vi "Test Open or Create.vi"(11 "Test Case In":refnum<class "Test Open Xml.lvclass">) -> (0 "error out":errorcluster, 3 "Test Case Out":refnum<class "Test Open Xml.lvclass">)   [LabVIEW 2020, in "Test Open Xml.lvclass"]
uses:
  Test Open Xml.lvclass
  C:/Program Files/National Instruments/LabVIEW 2025/vi.lib/Astemes/LUnit/Test Case.lvclass
  <vilib>/Astemes/LUnit/Test Case.lvclass/Test Case.ctl
  2c4bb252-386c-45a5-bd4c-bbe84a65a97e.vi
  <vilib>/Astemes/LUnit/Core/LUnit Test Case/Private/Append Pass Result.vi
  <vilib>/Astemes/LUnit/Core/LUnit Test Case/Private/Append Fail Result.vi
  2c4bb252-386c-45a5-bd4c-bbe84a65a97e.vi/9c5d11cd-9439-4240-a1ee-d9baace9c924.vi
  <vilib>/Astemes/LUnit/Core/LUnit Test Case/Private/Run In UI.vi
  <vilib>/Utility/error.llb/Clear Errors.vi
  Source/Open Xml.lvlib
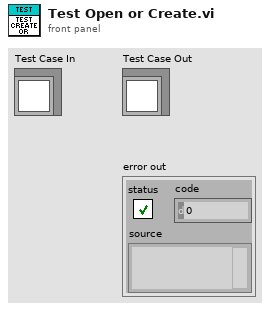
[diagram p1: front panel]
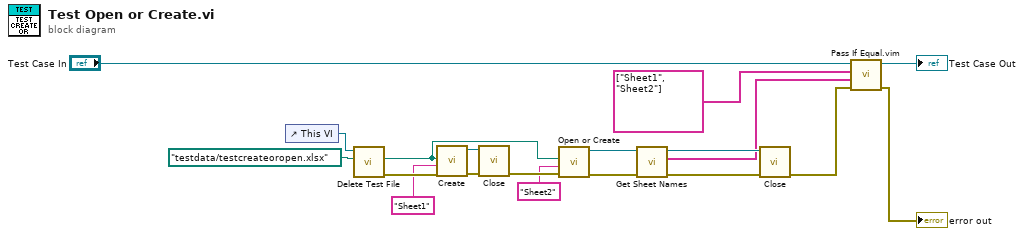
[diagram p0: block diagram]
diagram:
  n1 = control-ref of="This VI"() -> (w16:refnum<vi>)
  n2 = call "Delete Test File.vi"("name or relative path"=path "testdata/testcreateoropen.xlsx", "VI in"=w16) -> ("error out"=w12:errorcluster, "deleted path"=w10:path)  [unwired: 8 in]
  n3 = call "Create.vi"("error in"=w12, "SheetName"="Sheet1", "Path"=w10) -> ("error out"=w8:errorcluster, "SpreadsheetDoc"=w9:refnum<k24>)  [unwired: 7 in]
  n4 = call "Close.vi"("error in"=w8, "SpreadsheetDoc"=w9) -> ("error out"=w7:errorcluster)  [unwired: 9 in]
  n5 = call "Open or Create.vi"("error in"=w7, "SheetName"="Sheet2", "Path"=w10) -> ("error out"=w13:errorcluster, "SpreadsheetDoc"=w4:refnum<k24>)  [unwired: 7 in]
  n6 = call "Get Sheet Names.vi"("error in"=w13, "SpreadsheetDoc in"=w4) -> ("error out"=w5:errorcluster, "Sheet Names"=w1:string[], "SpreadsheetDoc out"=w3:refnum<k24>)  [unwired: 7 in]
  n7 = call "Close.vi"("error in"=w5, "SpreadsheetDoc"=w3) -> ("error out"=w14:errorcluster)  [unwired: 9 in]
  n8 = call "Pass If Equal.vim"("error in (no error)"=w14, "Actual"=w1, "Expected"=string[] ["Sheet1", "Sheet2"] ("Sheet Names"), "LUnit Test Case In"="Test Case In") -> ("error out"=→"error out":errorcluster, "LUnit Test Case Out"=→"Test Case Out":refnum<class "Test Open Xml.lvclass">)  [unwired: 6 in]
